vi "Example_OE2031&OE2041 Control.vi"() -> ()   [LabVIEW 2011]
uses:
  <vilib>/Utility/error.llb/DialogType.ctl
panel:
  in  "Sample count":u32
  out "Zero Data?":bool
  in  "buffer":u8
  out "Queue out":errorcluster caption="error out"
  out "Queue output":refnum<queue>
  in  "IP Address":string
  in  "Timeout":u32=100
  in  "Port":u32=10001
  out "Gain Overlaod":bool
  in  "Remote Mode":u16(ring) items=["USB"=0, "RS232"=1, "Ethernet"=3]
  out "Freq":dbl
  out "xita":dbl
  out "R":dbl
  out "Input Overlaod":bool
  out "PLL Lock":bool
  out "Error":string
  out "Serial Versions":string
  in  "Table":T1(tab) caption="选项卡控件"
  in  "OE2041_Configure Input Filter":T2 {"Input Impedance" items=["50Ω", "10MΩ"]; "Input Coupling" items=["AC", "DC"]; "Input Shield Grounding" items=["Float", "Ground"]; "Input Source" items=["A", "B"]}
  in  "OE2041_Configure Ref Phase":T3={"Reference Source"=0, "Sweep Mode"=0, "Start Frequency"=1000.0, "Stop Frequency"=5000.0, "Linear Step Frequency"=1000.0, "Log Step Percent"=10.0, "Step Time(ms)"=1000, "Sweep Run Mode"=0, "Internal Frequency"=1000.0, "Phase  (degree)"=0.0, "External Ref Trigger"=0, "Instrument Mode "=8} {"Instrument Mode" items=["OE2031-10M"=6, "OE2041-30M"=7, "OE2041-60M"=8]; "External Ref Trigger" items=["TTL Rising Edge", "Sine Zero Crossing"]; "Phase  (degree)" min=-180.0 max=180.0 format="%#.2g"; "Internal Frequency" min=1e-05 max=60000000.0 format="%#.3f"; "Sweep Run Mode" items=["Stop", "Singal", "Loop"]; "Log Step Percent" min=-100.0 max=100.0 format="%#.2f"; "Linear Step Frequency" min=1e-05 max=60000000.0 format="%#.3f"; "Stop Frequency" min=1e-05 max=60000000.0 format="%#.3f"; "Start Frequency" min=1e-05 max=60000000.0 format="%#.3f"; "Sweep Mode" items=["Linear", "Log"]; "Reference Source" items=["External", "Internal", "Internal Sweep", "Self"]}
  in  "OE2041_Configure Sens and Filter":T4={"Input Range"=0, "Sensitivity "=24, "Time Constant "=20, "Low Pass Filter Slope "=3, "Enable Sync Filter "=0} {"Enable Sync Filter" items=["OFF", "ON"]; "Low Pass Filter Slope" items=["6 dB/oct", "12 dB/oct", "18 db/oct", "24 dB/oct", "30 dB/oct", "36 dB/oct", "42 dB/oct", "48 dB/oct"]; "Time Constant" items=["30 ns", "60 ns", "125 ns", "250 ns", "500 ns", "1 us", "2 us", "4 us", "8 us", "16 us", "32 us", "64 us", "125 us", "250 us", "500 us", "1 ms", "2 ms", "4 ms", "8 ms", "16 ms", "32 ms", "65 ms", "125 ms", "250 ms", "500 ms", "1 s", "2 s", "4 s", "8 s", "17 s", "35 s", "70 s", "140 s", "275 s", "550 s", "1100 s", "2200 s", "4400 s"]; "Sensitivity" items=["1 nV/fA", "2 nV/fA", "5 nV/fA", "10 nV/fA", "20 nV/fA", "50 nV/fA", "100 nV/fA", "200 nV/fA", "500 nV/fA", "1 uV/pA", "2 uV/pA", "5 uV/pA", "10 uV/pA", "20 uV/pA", "50 uV/pA", "100 uV/pA", "200 uV/pA", "500 uV/pA", "1 mV/nA", "2 mV/nA", "5 mV/nA", "10 mV/nA", "20 mV/nA", "50 mV/nA", "100 mV/nA", "200 mV/nA", "500 mV/nA", "1 V/uA"]; "Input Range" items=["1V", "200mV", "50mV", "10mV", "2mV", "400uV"]}
  in  "OE2041_Configure Channel Out":T5={"parameter"=0, "Speed"=0, "Offset(%)"=0.0, "Expand"=1.0, "AUX OUT"=1.0, "Channel"=0} {"Channel" items=["CH1", "CH2", "CH3", "CH4"]; "AUX OUT" min=-10.0 max=10.0 format="%#.3g"; "Expand" min=1.0 max=256.0 format="%#_3g"; "Offset(%)" min=-100.0 max=100.0 format="%#_5g"; "Speed" items=["Slow", "Fast"]; "parameter" items=["AUXOUT", "X", "Y", "R", "Theta", "Xh1", "Yh1", "Rh1", "Theta h1", "Xh2", "Yh2", "Rh2", "Theta h2", "Xh3", "Yh3", "Rh3", "Theta h3", "X_Noise", "Y_Noise", "Frequency", "AUX-IN1", "AUX-IN2", "AUX-IN3", "AUX-IN4"]}
  in  "OE2041_Configure Sine Out":T6={"Start Value(V)"=0.1, "Sine Output Amplitude (V)"=1.0, "Stop Valve(V)"=1.0, "Sine Step Valve(V)"=0.1, "Step Time(ms) "=1000, "Sine Step Percent(%)"=10.0, "SineOut Mode"=0, "Sine Run Mode"=0, "ADD Mode"=0} {"ADD Mode" items=["OFF", "ON"]; "Sine Run Mode" items=["Stop", "Single", "Loop"]; "SineOut Mode" items=["OFF", "Fixed", "Linear", "Log"]; "Sine Step Percent(%)" min=0.0 max=100.0 format="%#.2g"; "Step Time(ms)" min=1 max=100000; "Sine Step Valve(V)" min=1e-06 max=1.0 format="%#.3g"; "Stop Valve(V)" min=1e-06 max=1.0 format="%#.3g"; "Sine Output Amplitude (V)" min=0.001 max=1.0 format="%#.3g"; "Start Value(V)" min=1e-06 max=1.0 format="%#.3g"}
  in  "OE2041_Configure Demodulator":T7={"A"=1, "F1"=1.0, "B"=1, "F2"=1.0, "Demodulator"=1, "Mode"=0, "Arbitrary Frequency"=1000.0, "Harmonic"=1, "Instrument Mode "=8} {"Instrument Mode" items=["OE2031-10M"=6, "OE2041-30M"=7, "OE2041-60M"=8]; "Harmonic" min=1 max=32767; "Arbitrary Frequency" min=1e-05 max=60000000.0 format="%#.3f"; "Mode" items=["Harm", "Arb_Freq", "Equation"]; "Demodulator" items=["1", "2", "3"]; "F2" min=1e-05 max=60000000.0 format="%#.3g"; "B" min=-32767; "F1" min=1e-05 max=60000000.0 format="%#.3g"; "A" min=-32767}
  in  "OE2041_Auto Setting":T8
  in  "Save Button":bool
  in  "file path":path
  in  "Sample Rate":dbl=0.1 min=0.001 max=100.0
  out "Status":string
  in  "Connect":bool
  in  "VISA resource name":refnum<visa-resource-name>
  in  "Baud Rate (921600)":u32=921600
  # "Tel          :   +86-020-84133345\nWebsite  :   www.ssi-instrument.com\nE-mail     :   support@si-instrument.com"
  # "E="
  # "×"
  # "+"
  # "×"
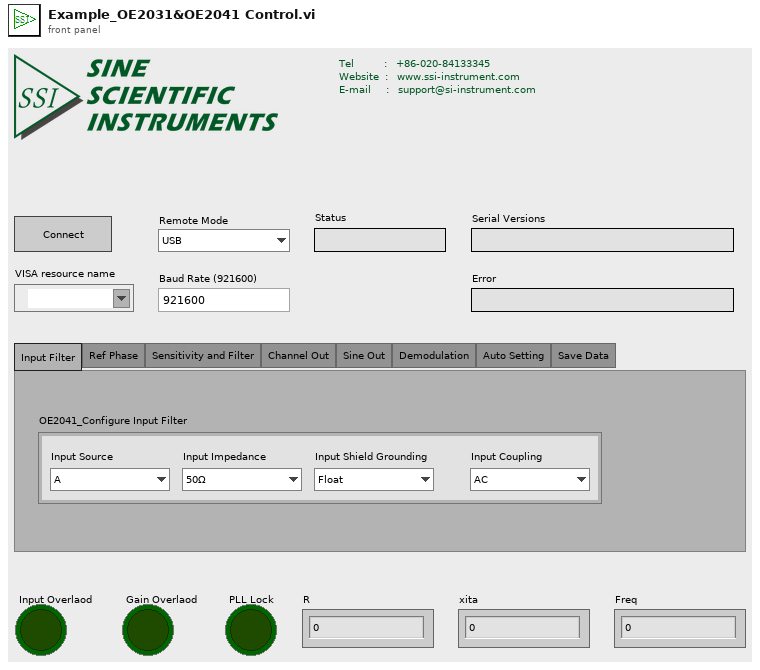
[diagram p1: front panel]
types:
  T1 = enum32{"Input Filter", "Ref Phase", "Sensitivity and Filter", "Channel Out", "Sine Out", "Demodulation", "Auto Setting", "Save Data"}
  T2 = cluster{"Input Source":u16, "Input Shield Grounding ":u16, "Input Coupling ":u16, "Input Impedance ":u16}
  T3 = cluster{"Reference Source":u16, "Sweep Mode":u16, "Start Frequency":dbl, "Stop Frequency":dbl, "Linear Step Frequency":dbl, "Log Step Percent":dbl, "Step Time(ms)":i32, "Sweep Run Mode":u16, "Internal Frequency":dbl, "Phase  (degree)":dbl, "External Ref Trigger":u16, "Instrument Mode ":u16}
  T4 = cluster{"Input Range":u16, "Sensitivity ":u16, "Time Constant ":u8, "Low Pass Filter Slope ":u8, "Enable Sync Filter ":u16}
  T5 = cluster{"parameter":u16, "Speed":u16, "Offset(%)":dbl, "Expand":dbl, "AUX OUT":dbl, "Channel":u16}
  T6 = cluster{"Start Value(V)":dbl, "Sine Output Amplitude (V)":dbl, "Stop Valve(V)":dbl, "Sine Step Valve(V)":dbl, "Step Time(ms) ":u32, "Sine Step Percent(%)":dbl, "SineOut Mode":u8, "Sine Run Mode":u8, "ADD Mode":u8}
  T7 = cluster{"A":i16, "F1":dbl, "B":i16, "F2":dbl, "Demodulator":u16, "Mode":u16, "Arbitrary Frequency":dbl, "Harmonic":u16, "Instrument Mode ":u16}
  T8 = cluster{"Auto Gain":bool, "Auto Phase":bool, "Auto Scale":bool}
  T9 = enum16{"OE1022", "OE1022D", "OE1201", "OE2031&OE2041", "OE1311&OE1351"}
  T10 = cluster{"Port":u32, "Timeout":u32, "IP Address":string}
  T11 = cluster{"PLL Lock(1: External Lock)":bool, "Input Overlaod":bool, "Gain Overlaod":bool}
  T12 = cluster{"X":dbl, "Y":dbl, "R":dbl, "θ":dbl, "Frequency":dbl, "XD1":dbl, "YD1":dbl, "RD1":dbl, "θD1":dbl, "XD2":dbl, "YD2":dbl, "RD2":dbl, "θD2":dbl, "XD3":dbl, "YD3":dbl, "RD3":dbl, "θD3":dbl, "X-Noise":dbl, "Y-Noise":dbl, "AUX-IN1":dbl, "AUX-IN2":dbl, "AUX-IN3":dbl, "AUX-IN4":dbl}
  T13 = typedef "DialogType.ctl" = u16
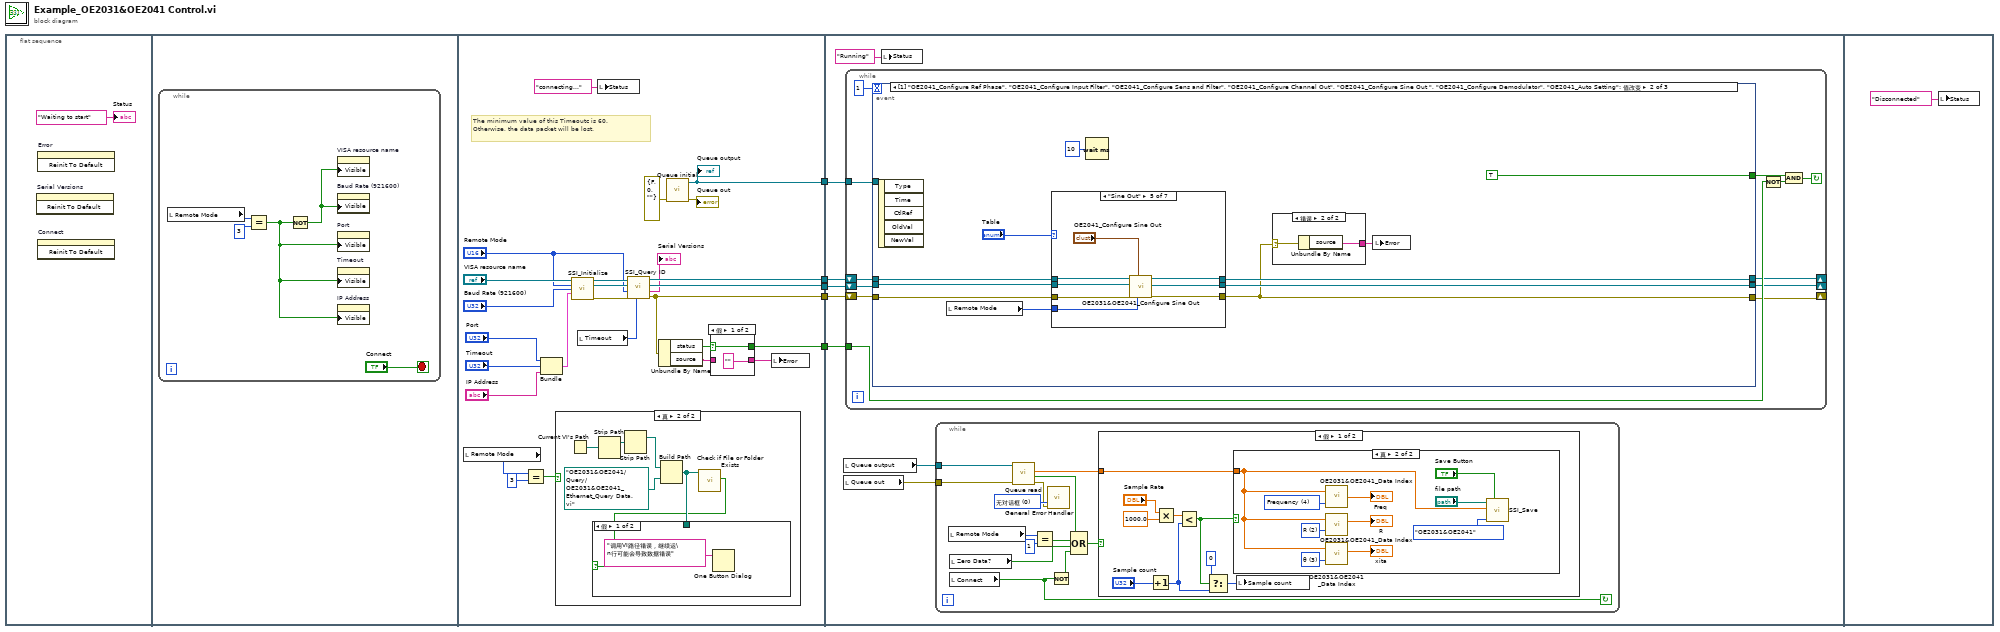
[diagram p0: block diagram]
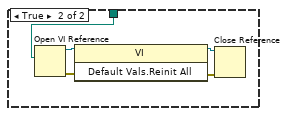
[diagram p3: hidden frame]
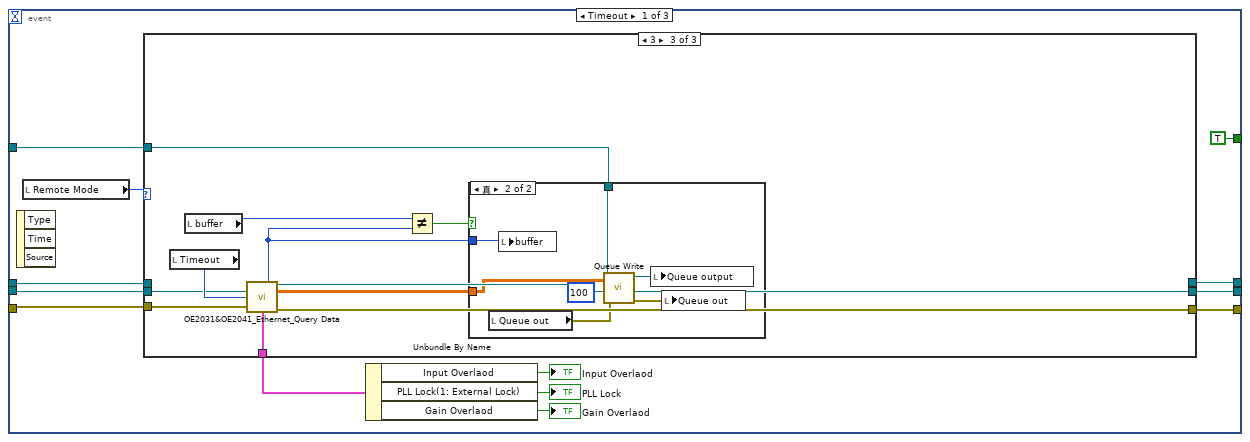
[diagram p7: hidden frame]
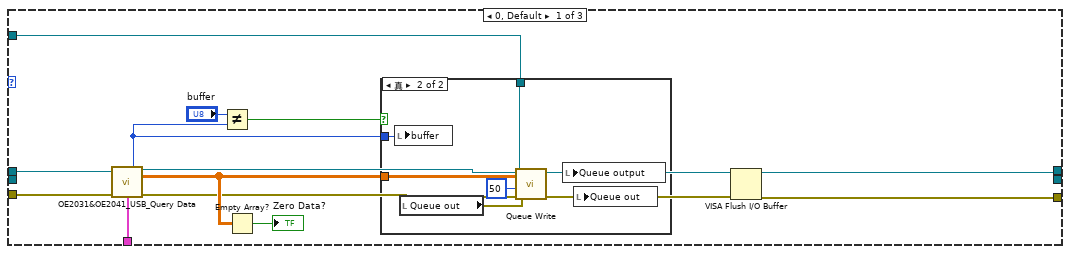
[diagram p8: hidden frame]
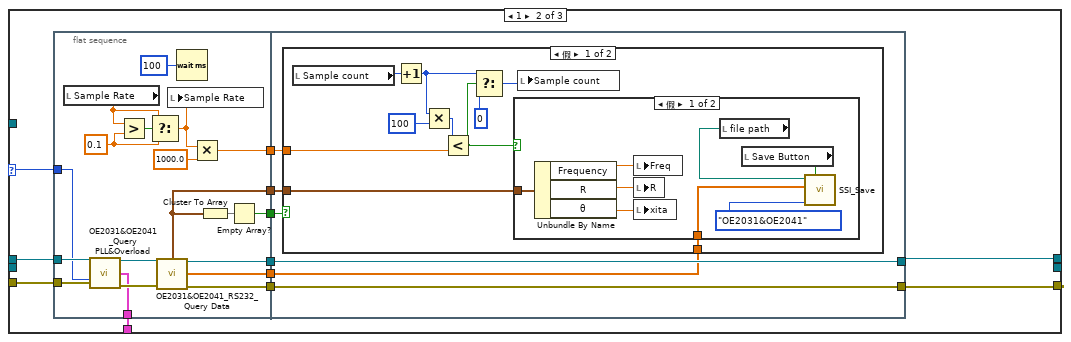
[diagram p10: hidden frame]
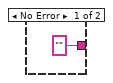
[diagram p14: hidden frame]
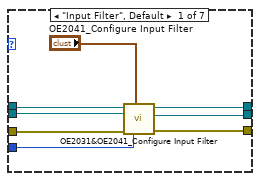
[diagram p15: hidden frame]
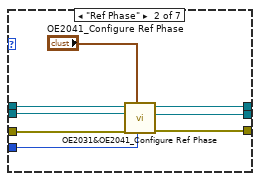
[diagram p16: hidden frame]
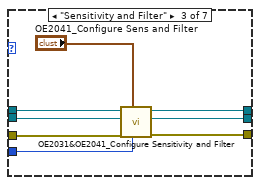
[diagram p17: hidden frame]
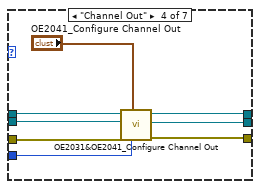
[diagram p18: hidden frame]
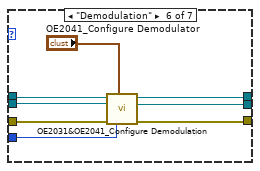
[diagram p19: hidden frame]
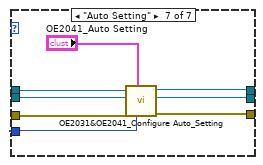
[diagram p20: hidden frame]
diagram:
  n1 = flat-sequence {
    tunnel: [w31] -> w5
    tunnel: [w30] -> w4
    tunnel: [w27] -> w3
    tunnel: [w24] -> w2
    tunnel: [w15] -> w1
    tunnel: w5 -> [w60]
    tunnel: w4 -> [w59]
    tunnel: w3 -> [w58]
    tunnel: w2 -> [w57]
    tunnel: w1 -> [w54]
    frame #0 {
      n2 = invoke on="Serial Versions" class="Str" method="Reinit To Default"() -> ()  [unwired: 3 in, 3 out]
      n3 = invoke on="Error" class="Str" method="Reinit To Default"() -> ()  [unwired: 3 in, 3 out]
      n4 = invoke on="Connect" class="Bool (严格)" method="Reinit To Default"() -> ()  [unwired: 3 in, 3 out]
      "Status" <- "Waiting to start" ("status")
    }
    frame #1 {
      n5 = while {
        stop <- "Connect" stop-if-true
        n6 = local read "Remote Mode"() -> (w10:u16)
        n7 = Equal?(x=w10, y=u16 3) -> (x = y?=w7:bool)
        n8 = Not(x=w7) -> (.not. x?=w8:bool)
        n9 = property on="VISA resource name" class="VISAName"("Visible"=w8) -> ()  [unwired: 2 in, 2 out]
        n10 = property on="Baud Rate (921600)" class="DigNum (严格)"("Visible"=w8) -> ()  [unwired: 2 in, 2 out]
        n11 = property on="Port" class="DigNum (严格)"("Visible"=w7) -> ()  [unwired: 2 in, 2 out]
        n12 = property on="Timeout" class="DigNum (严格)"("Visible"=w7) -> ()  [unwired: 2 in, 2 out]
        n13 = property on="IP Address" class="Str"("Visible"=w7) -> ()  [unwired: 2 in, 2 out]
      }
    }
    frame #2 {
      # "The minimum value of this Timeoutc is 60. \nOtherwise, the data packet will be lost."
      n14 = local read "Remote Mode"() -> (w14:u16)
      n15 = Equal?(x=w14, y=u16 3) -> (x = y?=w12:bool)
      n16 = Bundle("Port"="Port", "Timeout"="Timeout", "IP Address"="IP Address") -> (w19:T10)  [unwired: 1 in]
      n17 = case shown="真" w12 {
        frame False {
        }
        frame True {
          n18 = Current VI's Path() -> (path=w39:path)
          n19 = Strip Path(path=w39) -> (stripped path=w38:path)  [unwired: 1 out]
          n20 = Strip Path(path=w38) -> (stripped path=w40:path)  [unwired: 1 out]
          n21 = Build Path(base path=w40, name or relative path=path "OE2031&OE2041/Query/OE2031&OE2041_Ethernet_Query Data.vi") -> (appended path=w43:path)
          n22 = call <vilib>:"Check if File or Folder Exists.vi"("path"=w43) -> ("file or folder exists?"=w41:bool)  [unwired: 8 in, 2 out]
          n23 = case shown="假" w41 {
            tunnel: w43 -> [_ w49]
            frame False {
              n24 = One Button Dialog(message="调用VI路径错误，继续运\n行可能会导致数据错误" ("消息")) -> ()  [unwired: 1 in, 1 out]
            }
            frame True {
              n25 = Open VI Reference(vi path=w49) -> (vi reference=w46:refnum<vi>, error out=w45:errorcluster)  [unwired: 5 in]
              n26 = invoke class="VI" method="Default Vals.Reinit All"(reference=w46, error in=w45) -> (reference out=w48:refnum<vi>, error out=w47:errorcluster)  [unwired: 1 in, 1 out]
              n27 = Close Reference(reference=w48, error in (no error)=w47) -> ()  [unwired: 1 out]
            }
          }
        }
      }
      n28 = call "SSI_Initialize.vi"("VISA resource name"="VISA resource name", "Remote Mode"="Remote Mode", "baud rate (921600)"="Baud Rate (921600)", "Ethernet"=w19) -> ("VISA resource name out"=w35:refnum<visa-resource-name>, "connection ID(Ethernet)"=w34:refnum<k5>, "error out"=w33:errorcluster)  [unwired: 9 in]
      n29 = local read "Timeout"() -> (w18:u32)
      n30 = local write "Status"("connecting..." ("status")) -> ()
      n31 = call "SSI_Query ID.vi"("Timeout"=w18, "Error in (no error)"=w33, "Remote Mode"="Remote Mode", "Connection ID in"=w34, "VISA resource name"=w35) -> ("Error out"=w27:errorcluster, "Read Buffer"=→"Serial Versions":string, "Connection ID out"=w30:refnum<k5>, "VISA resource  out"=w31:refnum<visa-resource-name>)  [unwired: 3 in]
      n32 = Unbundle By Name(w27) -> ("status"=w26:bool, "source"=w25:string)
      n33 = call "Queue initial.vi"("Error in (no error)"=errorcluster {"status"=FALSE, "code"=0, "source"=""}) -> ("Error out"=→"Queue out":errorcluster, "Queue output"=w15:refnum<queue>)  [unwired: 9 in]
      "Queue output" <- w15
      n34 = case shown="假" w26 {
        selector: w26 -> [w51 w53]
        tunnel: [w51 w53] -> w24
        tunnel: ["" w52] -> w23
        tunnel: w25 -> [_ w52]
        frame False {
        }
        frame True {
        }
      }
      n35 = local write "Error"(w23) -> ()
    }
    frame #3 {
      n36 = local read "Queue output"() -> (w56:refnum<queue>)
      n37 = local read "Queue out"() -> (w55:errorcluster)
      n38 = while {
        tunnel: w57 -> [w101]
        tunnel: w54 -> [w97]
        shift-right: [w94] -> _
        shift-left: w58 -> [w98]
        shift-right: [w95] -> _
        shift-left: w59 -> [w99]
        shift-right: [w96] -> _
        shift-left: w60 -> [w100]
        stop <- w102 continue-if-true
        n39 = event shown="[1] \"OE2041_Configure Ref Phase\", \"OE2041_Configure Input Filter\", \"OE2041_Configure Sens and Filter\", \"OE2041_Configure Channel Out\", \"OE2041_Configure Sine Out \", \"OE2041_Configure Demodulator\", \"OE2041_Auto Setting\": 值改变" {
          selector: _ -> [_ _ _]
          dyn-events: _ -> [_ _ _]
          timeout: 1 -> [_ _ _]
          tunnel: [TRUE ("Stop") TRUE ("Stop") w282] -> w103
          tunnel: [w118 w213 w285] -> w94
          tunnel: [w117 w218 w284] -> w96
          tunnel: [w116 w217 w283] -> w95
          tunnel: w100 -> [w109 w221 w288]
          tunnel: w99 -> [w106 w220 w287]
          tunnel: w98 -> [w108 w219 w286]
          tunnel: w97 -> [w110 _ _]
          event Timeout {
            n40 = event-data() -> ()  [unwired: 1 in, 3 out]
            n41 = local read "Remote Mode"() -> (w114:u16)
            n42 = case shown="3" w114 {
              selector: w114 -> [_ w146 _]
              tunnel: [w122 w148 w202] -> w118
              tunnel: [w123 w147 _] -> w117
              tunnel: [_ _ w203] -> w116
              tunnel: w110 -> [w131 _ w201]
              tunnel: w109 -> [w121 w150 _]
              tunnel: w108 -> [w120 w149 w195]
              tunnel: [w119 w145 w194] -> w107
              tunnel: w106 -> [_ _ w196]
              frame 0, Default {
                n43 = call "OE2031&OE2041_USB_Query Data.vi"("VISA resource name"=w121, "Error in (no error)"=w120) -> ("Buffer Count"=w128:u8, "VISA resource  out"=w125:refnum<visa-resource-name>, "Total Data Array"=w127:dbl[][], "PLL&Overload"=w119:T11, "Error out"=w124:errorcluster)  [unwired: 6 in, 3 out]
                n44 = Not Equal?(x="buffer", y=w128) -> (x != y?=w129:bool)
                n45 = Empty Array?(array=w127) -> (empty?=→"Zero Data?":bool)
                n46 = case shown="真" w129 {
                  tunnel: w127 -> [_ w132]
                  tunnel: w131 -> [_ w137]
                  tunnel: w128 -> [_ w133]
                  frame False {
                  }
                  frame True {
                    n47 = local write "buffer"(w133) -> ()
                    n48 = local read "Queue out"() -> (w134:errorcluster)
                    n49 = call "Queue Write.vi"("Error in (no error)"=w134, "Group Count"=50, "Input Array"=w132, "Queue Input"=w137) -> ("Error out"=w135:errorcluster, "Queue output"=w136:refnum<queue>)  [unwired: 6 in]
                    n50 = local write "Queue output"(w136) -> ()
                    n51 = local write "Queue out"(w135) -> ()
                  }
                }
                n52 = VISA Flush I/O Buffer(VISA resource name=w125, error in (no error)=w124) -> (VISA resource name out=w123:refnum<visa-resource-name>, error out=w122:errorcluster)  [unwired: 1 in]
              }
              frame 1 {
                n53 = flat-sequence {
                  tunnel: [w159] -> w144
                  tunnel: [w160] -> w143
                  tunnel: [w164] -> w142
                  tunnel: [w163] -> w141
                  tunnel: [w158] -> w140
                  tunnel: [w157] -> w139
                  tunnel: [w152] -> w145
                  tunnel: w150 -> [w154]
                  tunnel: w149 -> [w155]
                  tunnel: w146 -> [w153]
                  tunnel: w144 -> [w174]
                  tunnel: w143 -> [w175]
                  tunnel: [w175] -> w147
                  tunnel: [w174] -> w148
                  tunnel: w142 -> [w171]
                  tunnel: w141 -> [w170]
                  tunnel: w140 -> [w172]
                  tunnel: w139 -> [w173]
                  frame #0 {
                    w167 = 0.1 ("y")
                    n54 = local read "Sample Rate"() -> (w162:dbl)
                    n55 = call "OE2031&OE2041_Query PLL&Overload.vi"("VISA resource name"=w154, "Remote Mode"=w153, "Error in (no error)"=w155) -> ("VISA resource  out"=w161:refnum<visa-resource-name>, "OE2041_Query PLL&Overload"=w152:T11, "Error out"=w156:errorcluster)  [unwired: 8 in, 2 out]
                    n56 = Greater?(x=w162, y=w167) -> (0:w166:bool)
                    n57 = Select(t=w162, s=w166, f=w167) -> (s? t:f=w165:dbl)
                    n58 = call "OE2031&OE2041_RS232_Query Data.vi"("VISA resource name"=w161, "Error in (no error)"=w156) -> ("VISA resource  out"=w160:refnum<visa-resource-name>, "Data Array"=w157:dbl[], "Parameter Values"=w158:T12, "Error out"=w159:errorcluster)  [unwired: 9 in, 1 out]
                    n59 = local write "Sample Rate"(w165) -> ()
                    n60 = Wait (ms)(milliseconds to wait=u32 100 ("等待时间（毫秒）")) -> ()  [unwired: 1 out]
                    n61 = Multiply(x=w165, y=1000.0) -> (x*y=w163:dbl)
                    n62 = Cluster To Array(cluster=w158) -> (array=w169:dbl[])
                    n63 = Empty Array?(array=w169) -> (empty?=w164:bool)
                  }
                  frame #1 {
                    n64 = case shown="假" w171 {
                      tunnel: w173 -> [w185 _]
                      tunnel: w172 -> [w184 _]
                      tunnel: w170 -> [w180 _]
                      frame False {
                        n65 = local read "Sample count"() -> (w183:u32)
                        n66 = Increment(x=w183) -> (x+1=w179:u32)
                        n67 = Multiply(x=w179, y=u32 100) -> (x*y=w181:u32)
                        n68 = Less?(x=w181, y=w180) -> (x < y?=w178:bool)
                        n69 = Select(t=w179, s=w178, f=0) -> (s? t:f=w177:u32)
                        n70 = case shown="假" w178 {
                          tunnel: w184 -> [w193 _]
                          tunnel: w185 -> [w189 _]
                          frame False {
                            n71 = Unbundle By Name(w193) -> ("Frequency"=w192:dbl, "R"=w191:dbl, "θ"=w190:dbl)
                            n72 = local write "Freq"(w192) -> ()
                            n73 = local write "R"(w191) -> ()
                            n74 = local write "xita"(w190) -> ()
                            n75 = local read "file path"() -> (w188:path)
                            n76 = local read "Save Button"() -> (w187:bool)
                            n77 = call "SSI_Save.vi"("file path (dialog if empty)"=w188, "1D data"=w189, "Instrument Mode"=T9."OE2031&OE2041", "Save Button"=w187) -> ()  [unwired: 7 in]
                          }
                          frame True {
                          }
                        }
                        n78 = local write "Sample count"(w177) -> ()
                      }
                      frame True {
                      }
                    }
                  }
                }
              }
              frame 3 {
                n79 = local read "Timeout"() -> (w204:u32)
                n80 = local read "buffer"() -> (w199:u8)
                n81 = call "OE2031&OE2041_Ethernet_Query Data.vi"("Connection ID in"=w196, "Timeout"=w204, "Error in (no error)"=w195) -> ("Buffer Count"=w198:u8, "Connection ID out"=w203:refnum<k5>, "Total Data Array"=w197:dbl[][], "PLL&Overload"=w194:T11, "Error out"=w202:errorcluster)  [unwired: 5 in, 3 out]
                n82 = Not Equal?(x=w199, y=w198) -> (x != y?=w200:bool)
                n83 = case shown="真" w200 {
                  tunnel: w201 -> [_ w210]
                  tunnel: w198 -> [_ w206]
                  tunnel: w197 -> [_ w205]
                  frame False {
                  }
                  frame True {
                    n84 = local read "Queue out"() -> (w207:errorcluster)
                    n85 = local write "buffer"(w206) -> ()
                    n86 = call "Queue Write.vi"("Error in (no error)"=w207, "Group Count"=100, "Input Array"=w205, "Queue Input"=w210) -> ("Error out"=w208:errorcluster, "Queue output"=w209:refnum<queue>)  [unwired: 6 in]
                    n87 = local write "Queue output"(w209) -> ()
                    n88 = local write "Queue out"(w208) -> ()
                  }
                }
              }
            }
            n89 = Unbundle By Name(w107) -> ("Input Overlaod"=→"Input Overlaod":bool, "PLL Lock(1: External Lock)"=→"PLL Lock":bool, "Gain Overlaod"=→"Gain Overlaod":bool)
          }
          event "OE2041_Configure Ref Phase", "OE2041_Configure Input Filter", "OE2041_Configure Sens and Filter", "OE2041_Configure Channel Out", "OE2041_Configure Sine Out", "OE2041_Configure Demodulator", "OE2041_Auto Setting": Value Change {
            n90 = event-data() -> ()  [unwired: 1 in, 5 out]
            n91 = local read "Remote Mode"() -> (w216:u16)
            n92 = case shown="\"Sine Out\"" "Table" {
              tunnel: w221 -> [w232 w241 w249 w254 w261 w270 w281]
              tunnel: w220 -> [w231 w240 w247 w255 w260 w271 w280]
              tunnel: w219 -> [w233 w239 w248 w257 w265 w273 w279]
              tunnel: [w228 w238 w245 w251 w262 w269 w277] -> w218
              tunnel: [w229 w237 w246 w253 w264 w268 w275] -> w213
              tunnel: [w230 w236 w244 w252 w263 w267 w276] -> w217
              tunnel: w216 -> [w227 w235 w243 w256 w259 w272 w278]
              frame "Input Filter", Default {
                n93 = call "OE2031&OE2041_Configure Input Filter.vi"("OE2041_Configure Input Filter"="OE2041_Configure Input Filter", "Error in (no error)"=w233, "Remote Mode"=w227, "Connection ID in"=w231, "VISA resource name"=w232) -> ("Error out"=w229:errorcluster, "Connection ID out"=w230:refnum<k5>, "VISA resource  out"=w228:refnum<visa-resource-name>)  [unwired: 3 in, 1 out]
              }
              frame "Ref Phase" {
                n94 = call "OE2031&OE2041_Configure Ref Phase.vi"("OE2041_Configure Ref Phase"="OE2041_Configure Ref Phase", "Error in (no error)"=w239, "Remote Mode"=w235, "Connection ID in"=w240, "VISA resource name"=w241) -> ("Error out"=w237:errorcluster, "Connection ID out"=w236:refnum<k5>, "VISA resource  out"=w238:refnum<visa-resource-name>)  [unwired: 3 in, 1 out]
              }
              frame "Sensitivity and Filter" {
                n95 = call "OE2031&OE2041_Configure Sensitivity and Filter.vi"("OE2041_Configure \nSens and Filter"="OE2041_Configure Sens and Filter", "Error in (no error)"=w248, "Remote Mode"=w243, "Connection ID in"=w247, "VISA resource name"=w249) -> ("Error out"=w246:errorcluster, "Connection ID out"=w244:refnum<k5>, "VISA resource  out"=w245:refnum<visa-resource-name>)  [unwired: 3 in, 1 out]
              }
              frame "Channel Out" {
                n96 = call "OE2031&OE2041_Configure Channel Out.vi"("OE2041_Configure Channel Out"="OE2041_Configure Channel Out", "Error in (no error)"=w257, "Remote Mode"=w256, "Connection ID in"=w255, "VISA resource name"=w254) -> ("Error out"=w253:errorcluster, "Connection ID out"=w252:refnum<k5>, "VISA resource  out"=w251:refnum<visa-resource-name>)  [unwired: 3 in, 1 out]
              }
              frame "Sine Out" {
                n97 = call "OE2031&OE2041_Configure Sine Out.vi"("OE2041_Configure Sine Out"="OE2041_Configure Sine Out", "Error in (no error)"=w265, "Remote Mode"=w259, "Connection ID in"=w260, "VISA resource name"=w261) -> ("Error out"=w264:errorcluster, "Connection ID out"=w263:refnum<k5>, "VISA resource  out"=w262:refnum<visa-resource-name>)  [unwired: 3 in, 1 out]
              }
              frame "Demodulation" {
                n98 = call "OE2031&OE2041_Configure Demodulation.vi"("OE2041_Configure Demodulator"="OE2041_Configure Demodulator", "Error in (no error)"=w273, "Remote Mode"=w272, "Connection ID in"=w271, "VISA resource name"=w270) -> ("Error out"=w268:errorcluster, "Connection ID out"=w267:refnum<k5>, "VISA resource  out"=w269:refnum<visa-resource-name>)  [unwired: 3 in, 1 out]
              }
              frame "Auto Setting" {
                n99 = call "OE2031&OE2041_Configure Auto_Setting.vi"("OE2041_Auto Setting"="OE2041_Auto Setting", "Error in (no error)"=w279, "Remote Mode"=w278, "Connection ID in"=w280, "VISA resource name"=w281) -> ("Error out"=w275:errorcluster, "Connection ID out"=w276:refnum<k5>, "VISA resource  out"=w277:refnum<visa-resource-name>)  [unwired: 3 in, 1 out]
              }
            }
            n100 = Wait (ms)(milliseconds to wait=u32 10 ("等待时间（毫秒）")) -> ()  [unwired: 1 out]
            n101 = case shown="错误" w213 {
              selector: w213 -> [_ w225]
              tunnel: ["" ("source") w224] -> w214
              frame No Error {
              }
              frame Error {
                n102 = Unbundle By Name(w225) -> ("source"=w224:string)
              }
            }
            n103 = local write "Error"(w214) -> ()
          }
          event "Connect": Value Change {
            n104 = event-data() -> ("NewVal"=w282:bool)  [unwired: 1 in, 4 out]
            n105 = case shown="假" w282 {
              tunnel: w288 -> [w293 w298]
              tunnel: w287 -> [w292 w297]
              tunnel: w286 -> [w291 w299]
              tunnel: [w290 w299] -> w285
              tunnel: [_ w298] -> w284
              tunnel: [_ w297] -> w283
              frame False {
                n106 = call "SSI_Close.vi"("Error in (no error)"=w291, "Connection ID in"=w292, "VISA resource name"=w293) -> ("Error out"=w290:errorcluster)  [unwired: 4 in]
                n107 = case shown="无错误" w290 {
                  selector: w290 -> [_ w296]
                  tunnel: ["Correct Connection!No Error..." ("source") w295] -> w289
                  frame No Error {
                  }
                  frame Error {
                    n108 = Unbundle By Name(w296) -> ("source"=w295:string)
                  }
                }
                "Error" <- w289
              }
              frame True {
              }
            }
          }
        }
        n109 = Not(x=w101) -> (.not. x?=w104:bool)
        n110 = And(x=w103, y=w104) -> (x .and. y?=w102:bool)
      }
      n111 = local write "Status"("Running" ("status")) -> ()
      n112 = while {
        tunnel: w56 -> [w67]
        tunnel: w55 -> [w66]
        stop <- w62 continue-if-true
        w69 = T13 0 items=["无对话框", "确定信息", "继续或停止信息", "确定信息＋警告", "继续/停止+警告"] ("type of dialog (OK msg:1)")
        n113 = local read "Remote Mode"() -> (w74:u16)
        n114 = local read "Zero Data?"() -> (w70:bool)
        n115 = local read "Connect"() -> (w62:bool)
        n116 = call "Queue read.vi"("Error in (no error)"=w66, "Queue Input"=w67) -> ("Error out"=w68:errorcluster, "Timeout？"=w64:bool, "Output Array"=w65:sgl[])  [unwired: 7 in]
        n117 = Equal?(x=w74, y=u16 1) -> (x = y?=w71:bool)
        n118 = call <vilib>:"General Error Handler.vi"("type of dialog (OK msg:1)"=w69, "error in (no error)"=w68) -> ()  [unwired: 9 in, 5 out]
        n119 = Not(x=w62) -> (.not. x?=w63:bool)
        n120 = Compound Arithmetic op=OR(w64, w71, w70, w63) -> (w72:bool)
        n121 = case shown="假" w72 {
          tunnel: w65 -> [w83 _]
          frame False {
            n122 = Increment(x="Sample count") -> (x+1=w77:u32)
            n123 = Multiply(x="Sample Rate", y=1000.0) -> (x*y=w81:dbl)
            n124 = Less?(x=w81, y=w77) -> (x < y?=w78:bool)
            n125 = Select(t=0, s=w78, f=w77) -> (s? t:f=w76:u32)
            n126 = case shown="真" w78 {
              tunnel: w83 -> [_ w85]
              frame False {
              }
              frame True {
                w93 = u16 3 items=["X", "Y", "R", "θ", "Frequency", "XD1", "YD1", "RD1", "θD1", "XD2", "YD2", "RD2", "θD2", "XD3", "YD3", "RD3", "θD3", "X_Noise", "Y_Noise", "AUXADC1", "AUXADC2", "AUXADC3", "AUXADC4"] ("Parameter Type")
                w92 = u16 2 items=["X", "Y", "R", "θ", "Frequency", "XD1", "YD1", "RD1", "θD1", "XD2", "YD2", "RD2", "θD2", "XD3", "YD3", "RD3", "θD3", "X_Noise", "Y_Noise", "AUXADC1", "AUXADC2", "AUXADC3", "AUXADC4"] ("Parameter Type")
                w91 = u16 4 items=["X", "Y", "R", "θ", "Frequency", "XD1", "YD1", "RD1", "θD1", "XD2", "YD2", "RD2", "θD2", "XD3", "YD3", "RD3", "θD3", "X_Noise", "Y_Noise", "AUXADC1", "AUXADC2", "AUXADC3", "AUXADC4"] ("Parameter Type")
                n127 = call "OE2031&OE2041_Data Index.vi"("Parameter Type"=w91, "Input Date Array"=w85) -> ("Parameter"=→"Freq":dbl)
                n128 = call "OE2031&OE2041_Data Index.vi"("Parameter Type"=w92, "Input Date Array"=w85) -> ("Parameter"=→"R":dbl)
                n129 = call "OE2031&OE2041_Data Index.vi"("Parameter Type"=w93, "Input Date Array"=w85) -> ("Parameter"=→"xita":dbl)
                n130 = call "SSI_Save.vi"("file path (dialog if empty)"="file path", "1D data"=w85, "Instrument Mode"=T9."OE2031&OE2041", "Save Button"="Save Button") -> ()  [unwired: 7 in]
              }
            }
            n131 = local write "Sample count"(w76) -> ()
          }
          frame True {
          }
        }
      }
    }
    frame #4 {
      n132 = local write "Status"("Disconnected" ("status")) -> ()
    }
  }
